vi "TestClient.vi"() -> ()   [LabVIEW 2019]
panel:
  out "value 4":u8[](array[numeric])
  out "value 3":u8[](array[numeric])
  out "value 2":u8[](array[numeric])
  out "value":i32
  out "Data Out":u8[](array[numeric])
  in  "stop":bool
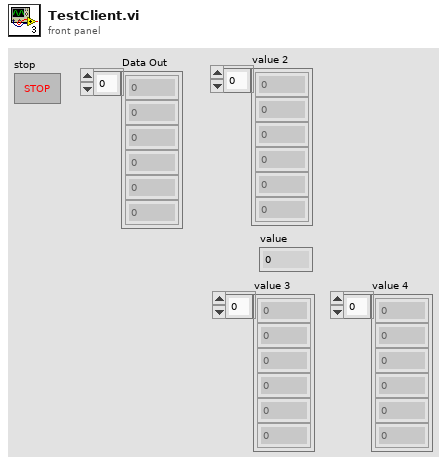
[diagram p1: front panel]
types:
  T1 = enum16{"big-endian, network order", "native, host order", "little-endian"}
  T2 = enum16{"Standard", "Buffered", "CRLF", "Immediate"}
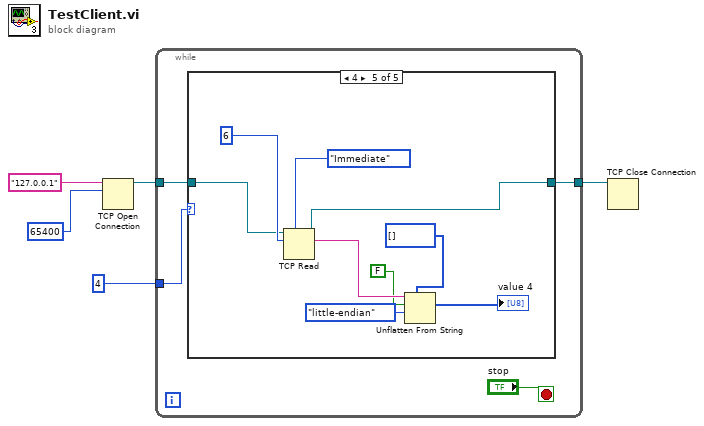
[diagram p0: block diagram]
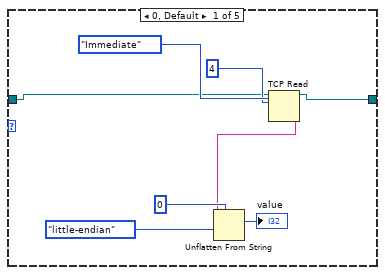
[diagram p2: hidden frame]
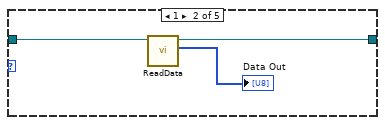
[diagram p3: hidden frame]
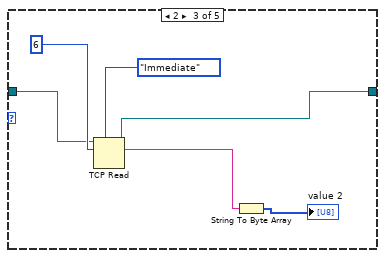
[diagram p4: hidden frame]
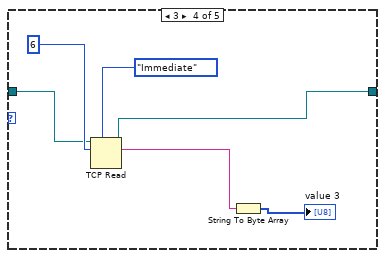
[diagram p5: hidden frame]
diagram:
  n1 = TCP Open Connection(address="127.0.0.1", remote port or service name=65400 ("port")) -> (connection ID=w3:refnum<k5>)  [unwired: 3 in, 1 out]
  n2 = while {
    tunnel: w3 -> [w9]
    tunnel: [w7] -> w2
    tunnel: 4 -> [w6]
    stop <- "stop" stop-if-true
    n3 = case shown="4" w6 {
      tunnel: w9 -> [w15 w20 w25 w28 w39]
      tunnel: [w14 w19 w24 w27 w38] -> w7
      frame 0, Default {
        n4 = TCP Read(connection ID=w15, bytes to read=4, 7:T2."Immediate" ("mode (standard)")) -> (connection ID out=w14:refnum<k5>, data out=w12:string)  [unwired: 2 in, 1 out]
        n5 = Unflatten From String(type=0, binary string=w12, byte order (0:big-endian, network order)=T1."little-endian") -> (value=→"value":i32)  [unwired: 2 in, 2 out]
      }
      frame 1 {
        n6 = call "ReadData.vi"("Connection In"=w20) -> ("Data Out"=→"Data Out":u8[], "Connection Out"=w19:refnum<k5>)  [unwired: 8 in, 1 out]
      }
      frame 2 {
        n7 = TCP Read(connection ID=w25, bytes to read=6 ("dimension size"), 7:T2."Immediate" ("mode (standard)")) -> (connection ID out=w24:refnum<k5>, data out=w23:string)  [unwired: 2 in, 1 out]
        n8 = String To Byte Array(string=w23) -> (unsigned byte array=→"value 2":u8[])
      }
      frame 3 {
        n9 = TCP Read(connection ID=w28, bytes to read=6 ("dimension size"), 7:T2."Immediate" ("mode (standard)")) -> (connection ID out=w27:refnum<k5>, data out=w31:string)  [unwired: 2 in, 1 out]
        n10 = String To Byte Array(string=w31) -> (unsigned byte array=→"value 3":u8[])
      }
      frame 4 {
        n11 = TCP Read(connection ID=w39, bytes to read=6 ("dimension size"), 7:T2."Immediate" ("mode (standard)")) -> (connection ID out=w38:refnum<k5>, data out=w35:string)  [unwired: 2 in, 1 out]
        n12 = Unflatten From String(type=u8[] [], binary string=w35, data includes array or string size? (T)=FALSE, byte order (0:big-endian, network order)=T1."little-endian") -> (value=→"value 4":u8[])  [unwired: 1 in, 2 out]
      }
    }
  }
  n13 = TCP Close Connection(connection ID=w2) -> ()  [unwired: 2 in, 2 out]
